vi "counter 2 with semaphore.vi"() -> ()   [LabVIEW 2010]
panel:
  out "전체 \n카운트":i32 caption="전체 카운트"
  out "카운트 2":i32
  out "진행 중 합계":i32
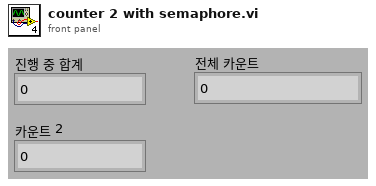
[diagram p1: front panel]
types:
  T1 = typedef "Semaphore RefNum" = refnum<k1>
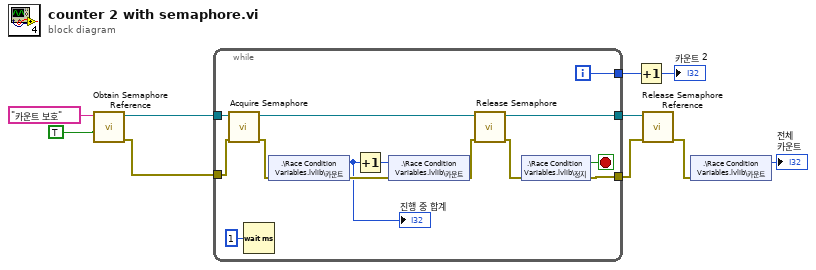
[diagram p0: block diagram]
diagram:
  n1 = call <vilib>:"Obtain Semaphore Reference.vi"("create if not found (T)"=TRUE ("return existing (F)"), "name (unnamed)"="카운트 보호") -> ("error out"=w4:errorcluster, "semaphore"=w5:T1)  [unwired: 3 in, 1 out]
  n2 = while {
    tunnel: [w23] -> w10
    tunnel: w4 -> [w17]
    tunnel: [w22] -> w2
    tunnel: w5 -> [w18]
    tunnel: [w11] -> w3
    i -> [w23]
    stop <- w12 stop-if-true
    n3 = call <vilib>:"Acquire Semaphore.vi"("error in (no error)"=w17, "semaphore"=w18) -> ("error out"=w16:errorcluster, "semaphore out"=w13:T1)  [unwired: 3 in, 1 out]
    n4 = Wait (ms)(milliseconds to wait=u32 1) -> ()  [unwired: 1 out]
    n5 = shared-variable ".\\Race Condition Variables.lvlib\\카운트"(error in=w16) -> (w19:i32, error out=w24:errorcluster)
    "진행 중 합계" <- w19
    n6 = Increment(x=w19) -> (x+1=w20:i32)
    n7 = shared-variable ".\\Race Condition Variables.lvlib\\카운트"(w20, error in=w24) -> (error out=w15:errorcluster)
    n8 = call <vilib>:"Release Semaphore.vi"("error in (no error)"=w15, "semaphore"=w13) -> ("error out"=w14:errorcluster, "semaphore out"=w11:T1)  [unwired: 4 in]
    n9 = shared-variable ".\\Race Condition Variables.lvlib\\정지"(error in=w14) -> (w12:bool, error out=w22:errorcluster)
  }
  n10 = Increment(x=w10) -> (x+1=→"카운트 2":i32)
  n11 = call <vilib>:"Release Semaphore Reference.vi"("error in (no error)"=w2, "semaphore"=w3) -> ("error out"=w1:errorcluster)  [unwired: 8 in, 1 out]
  n12 = shared-variable ".\\Race Condition Variables.lvlib\\카운트"(error in=w1) -> (→"전체 \n카운트":i32)  [unwired: 1 out]
